vi "ArmNetwork.vi"   [LabVIEW 2023]
uses:
  ArmNetworkingGlobal.vi
  <vilib>/Rock Robotics/Network Tables/NT Write Number.vi
  <vilib>/Rock Robotics/Network Tables/NT Write Boolean.vi
  ArmGlobal.vi
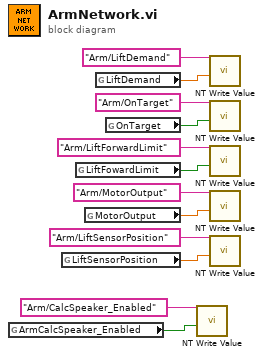
[diagram p0: block diagram]
diagram:
  n1 = global read "ArmGlobal.vi" "ArmCalcSpeaker_Enabled"() -> (w2:bool)
  n2 = global read "ArmNetworkingGlobal.vi" "LiftSensorPosition"() -> (w3:dbl)
  n3 = global read "ArmNetworkingGlobal.vi" "LiftFowardLimit"() -> (w7:bool)
  n4 = global read "ArmNetworkingGlobal.vi" "MotorOutput"() -> (w5:dbl)
  n5 = global read "ArmNetworkingGlobal.vi" "LiftDemand"() -> (w11:dbl)
  n6 = global read "ArmNetworkingGlobal.vi" "OnTarget"() -> (w9:bool)
  n7 = call-poly <vilib>:"NT Write Value.vi"("value"=w2, "name"="Arm/CalcSpeaker_Enabled") -> ()  [unwired: 9 in, 1 out]
  n8 = call-poly <vilib>:"NT Write Value.vi"("value"=w11, "name"="Arm/LiftDemand") -> ()  [unwired: 9 in, 1 out]
  n9 = call-poly <vilib>:"NT Write Value.vi"("value"=w9, "name"="Arm/OnTarget") -> ()  [unwired: 9 in, 1 out]
  n10 = call-poly <vilib>:"NT Write Value.vi"("value"=w7, "name"="Arm/LiftForwardLimit") -> ()  [unwired: 9 in, 1 out]
  n11 = call-poly <vilib>:"NT Write Value.vi"("value"=w5, "name"="Arm/MotorOutput") -> ()  [unwired: 9 in, 1 out]
  n12 = call-poly <vilib>:"NT Write Value.vi"("value"=w3, "name"="Arm/LiftSensorPosition") -> ()  [unwired: 9 in, 1 out]
